vi "ROI entry-ROI lines check and correct.vi"(9 "Old ROI file's data in":dbl[][](array[numeric]), 11 "New ROI file's data in in":dbl[][](array[numeric])) -> (1 "Final OK":bool, 2 "Mismatch":bool, 3 "New ROI file's data out":dbl[][](array[numeric]), 5 "Vertical?":bool[](array[boolean]))   [LabVIEW 2020]
panel:
  out "New number of lines":dbl[](array[numeric])
  out "Mismatch by (pixels)":dbl[](array[numeric])
  out "Mismatch":bool[](array[boolean])
  out "Equal to the first value?":bool[](array[boolean])
  out "Equal to the first value?":bool[](array[boolean])
  out "Old number of lines":dbl[](array[numeric])
  out "Old length":dbl[](array[numeric])
  out "Equal to the first value?":bool[](array[boolean])
  out "Equal to the first value?":bool[](array[boolean])
  out "New number of lines (equalised)":dbl[](array[numeric])
  out "New length":dbl[](array[numeric])
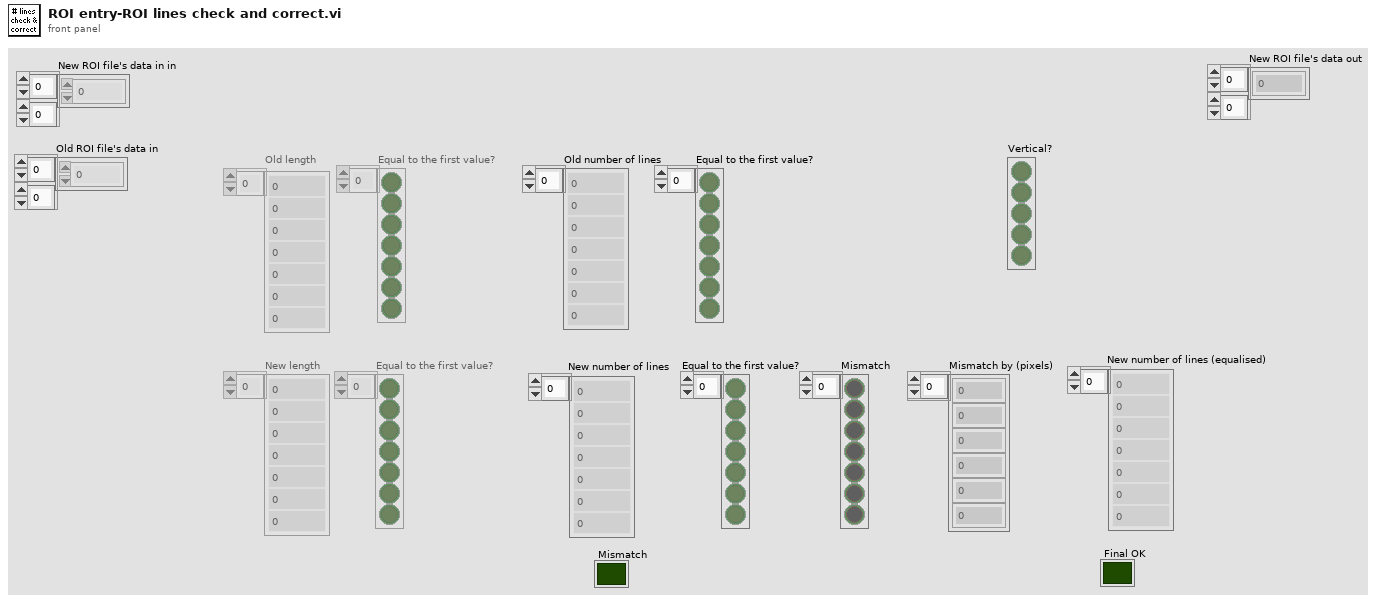
[diagram p1: front panel]
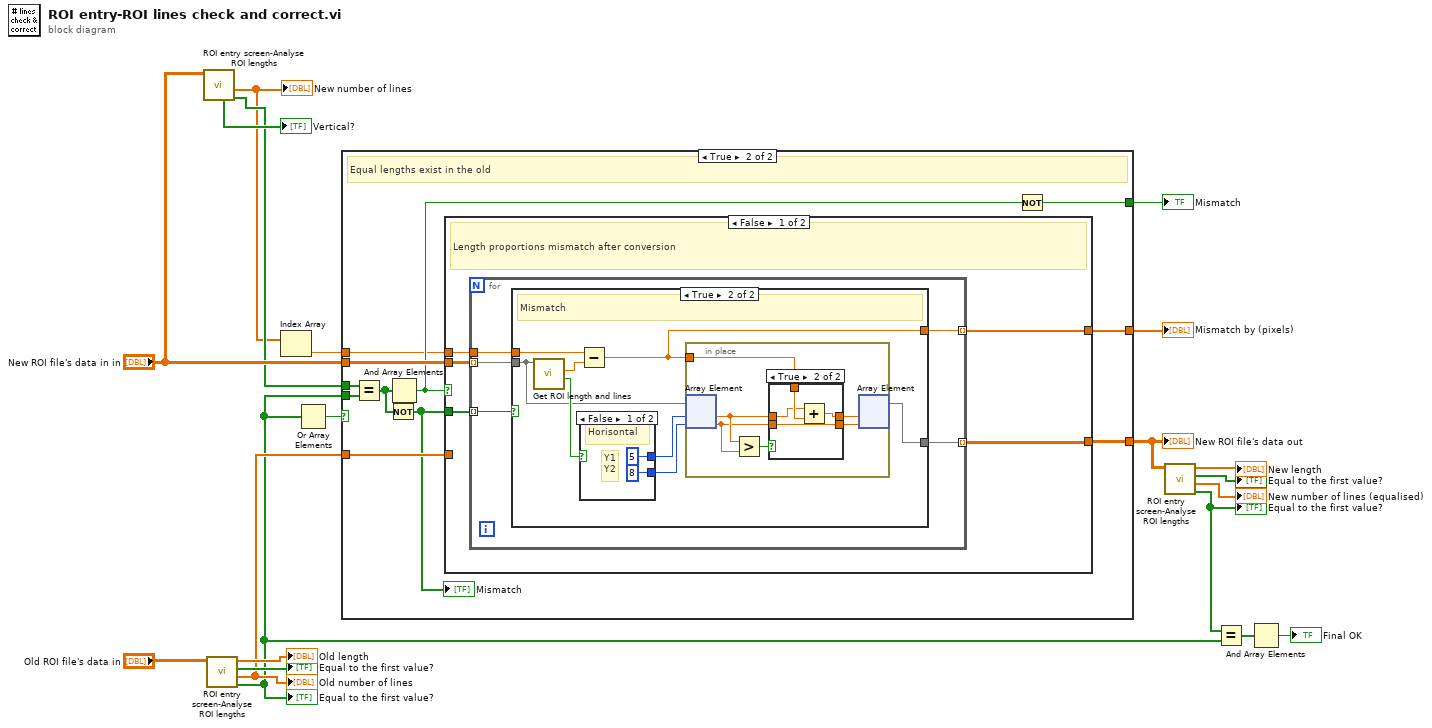
[diagram p0: block diagram]
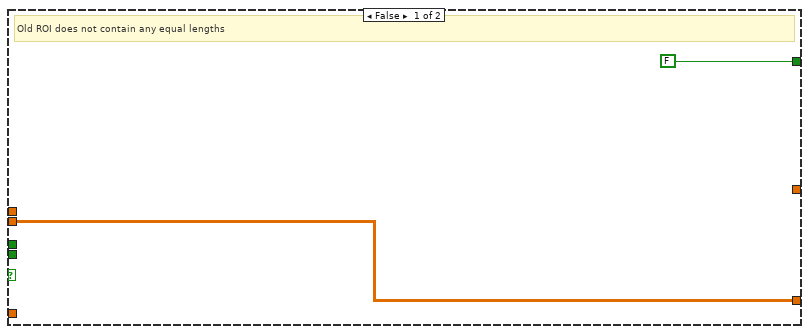
[diagram p2: hidden frame]
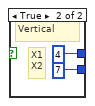
[diagram p4: hidden frame]
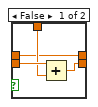
[diagram p5: hidden frame]
diagram:
  n1 = call "ROI entry screen-Analyse ROI lengths.vi"("Old ROI file's data in"="New ROI file's data in in") -> ("Lines-Equal to the first value?"=w16:bool[], "Number of lines []"=w6:dbl[], "Vertical?"=→"Vertical?":bool[])  [unwired: 6 in, 2 out]
  "New number of lines" <- w6
  n2 = call "ROI entry screen-Analyse ROI lengths.vi"("Old ROI file's data in"="Old ROI file's data in") -> ("Lines-Equal to the first value?"=w9:bool[], "Number of lines []"=w12:dbl[], "Lengths-Equal to the first value?"=→"Equal to the first value?":bool[], "Length []"=→"Old length":dbl[])  [unwired: 6 in, 1 out]
  "Old number of lines" <- w12
  "Equal to the first value?" <- w9
  n3 = Index Array(array=w6) -> (element=w20:dbl)  [unwired: 1 in]
  n4 = Or Array Elements(Boolean array=w9) -> (logical OR=w19:bool)
  n5 = case shown="True" w19 {
    tunnel: "New ROI file's data in in" -> [w22 w33]
    tunnel: w12 -> [_ w32]
    tunnel: [w22 w31] -> w11
    tunnel: [FALSE w24] -> w7
    tunnel: w20 -> [_ w28]
    tunnel: w16 -> [_ w27]
    tunnel: w9 -> [_ w26]
    tunnel: [_ w23] -> w1
    frame False {
      # "Old ROI does not contain any equal lengths"
    }
    frame True {
      # "Equal lengths exist in the old"
      n6 = Equal?(x=w27, y=w26) -> (x = y?=w29:bool[])
      n7 = Not(x=w29) -> (.not. x?=w25:bool[])
      "Mismatch" <- w25
      n8 = And Array Elements(Boolean array=w29) -> (logical AND=w30:bool)
      n9 = case shown="False" w30 {
        tunnel: w33 -> [w38 w71]
        tunnel: w32 -> [_ _]
        tunnel: [w35 w71] -> w31
        tunnel: w25 -> [w37 _]
        tunnel: w28 -> [w36 _]
        tunnel: [w34 _] -> w23
        frame False {
          # "Length proportions mismatch after conversion"
          n10 = for {
            tunnel: w38 -> [w42] mode=indexing
            tunnel: w37 -> [w43] mode=indexing
            tunnel: w36 -> [w40]
            tunnel: [w41] -> w35 mode=indexing
            tunnel: [w39] -> w34 mode=indexing
            n11 = case shown="True" w43 {
              tunnel: [w44 w45] -> w41
              tunnel: w42 -> [w44 w46]
              tunnel: w40 -> [_ w52]
              tunnel: [_ w50] -> w39
              frame False {
                # "OK"
              }
              frame True {
                # "Mismatch"
                n12 = call "Get ROI length and lines.vi"("Old ROI file's data in"=w46) -> ("Vertical"=w49:bool, "Number of lines"=w51:dbl)  [unwired: 8 in, 1 out]
                n13 = Subtract(x=w52, y=w51) -> (x-y=w50:dbl)
                n14 = case shown="False" w49 {
                  tunnel: [5 ("index") 4 ("index")] -> w48
                  tunnel: [8 ("index") 7 ("index")] -> w47
                  frame False {
                    # "Y1\nY2"
                    # "Horisontal"
                  }
                  frame True {
                    # "X1\nX2"
                    # "Vertical"
                  }
                }
                n15 = in-place {
                  in-place-border: w50 -> [w62]
                  n16 = in-place-array #1(w46, w48, w47) -> (w59:dbl, w57:dbl)
                  n17 = Greater?(x=w59, y=w57) -> (0:w60:bool)
                  n18 = case shown="True" w60 {
                    tunnel: w57 -> [w66 w68]
                    tunnel: w62 -> [w65 w70]
                    tunnel: [w64 w68] -> w61
                    tunnel: w59 -> [w63 w69]
                    tunnel: [w63 w67] -> w58
                    frame False {
                      n19 = Add(x=w66, y=w65) -> (x+y=w64:dbl)
                    }
                    frame True {
                      n20 = Add(x=w69, y=w70) -> (x+y=w67:dbl)
                    }
                  }
                  n21 = in-place-array #1(w58, w61) -> (w45:dbl[])  [unwired: 2 out]
                }
              }
            }
          }
        }
        frame True {
          # "Do nothing"
          # "Length proportions match after conversion"
        }
      }
      n22 = Not(x=w30) -> (.not. x?=w24:bool)
    }
  }
  "New ROI file's data out" <- w11
  "Mismatch" <- w7
  "Mismatch by (pixels)" <- w1
  n23 = call "ROI entry screen-Analyse ROI lengths.vi"("Old ROI file's data in"=w11) -> ("Lines-Equal to the first value?"=w2:bool[], "Number of lines []"=→"New number of lines (equalised)":dbl[], "Lengths-Equal to the first value?"=→"Equal to the first value?":bool[], "Length []"=→"New length":dbl[])  [unwired: 6 in, 1 out]
  "Equal to the first value?" <- w2
  n24 = Equal?(x=w2, y=w9) -> (x = y?=w10:bool[])
  n25 = And Array Elements(Boolean array=w10) -> (logical AND=→"Final OK":bool)
